vi "DeleteFileIfExisting.vi"(11 "filename":path) -> ()   [LabVIEW 2011]
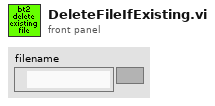
[diagram p1: front panel]
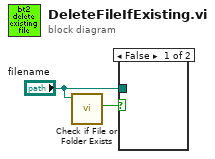
[diagram p0: block diagram]
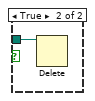
[diagram p2: hidden frame]
diagram:
  n1 = call <vilib>:"Check if File or Folder Exists.vi"("path"="filename") -> ("file or folder exists?"=w1:bool)  [unwired: 8 in, 2 out]
  n2 = case shown="False" w1 {
    tunnel: "filename" -> [_ w3]
    frame False {
    }
    frame True {
      n3 = Delete(path (use dialog)=w3) -> ()  [unwired: 4 in, 3 out]
    }
  }
